vi "Check Labels.vi"(6 "Labels":map{string, string}(c390), 11 "Histogram in":refnum<class "Histogram.lvclass">) -> (1 "Label Values":string[](array[string]), 2 "Valid Labels":bool, 3 "Samples":map{string, refnum<class "Sample.lvclass">}(c390))   [LabVIEW 2020, in "Metrics.lvlib" / "Histogram.lvclass"]
uses:
  Histogram.lvclass
  C:/Github-locals/PromVIEW/src/metrics/metric/Metric.lvclass
  sample/Sample.lvclass
  metric/Metric.lvclass/Metric.ctl
  metric/Read Samples.vi
  metric/Read Label Names.vi
  Histogram.lvclass/Histogram.ctl
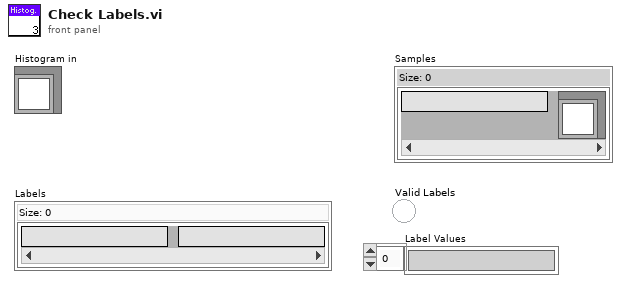
[diagram p1: front panel]
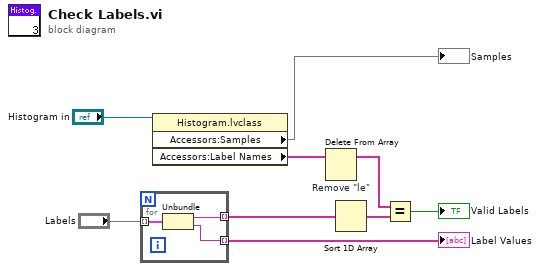
[diagram p0: block diagram]
diagram:
  n1 = for {
    tunnel: [w12] -> w7 mode=indexing
    tunnel: [w11] -> w4 mode=indexing
    tunnel: "Labels" -> [w10] mode=indexing
    n2 = Unbundle(w10) -> ("labelname"=w12:string, "labelvalue"=w11:string)
  }
  "Label Values" <- w4
  n3 = property class="Histogram.lvclass"(reference="Histogram in") -> ("Accessors:Samples"=→"Samples":map{string, refnum<class "Sample.lvclass">}, "Accessors:Label Names"=w2:string[])  [unwired: 1 in, 2 out]
  n4 = Delete From Array "Remove \"le\""(array=w2) -> (array with subset deleted=w5:string[])  [unwired: 2 in, 1 out]
  n5 = Sort 1D Array(array=w7) -> (sorted array=w9:string[])
  n6 = Equal?(x=w5, y=w9) -> (x = y?=→"Valid Labels":bool)
